vi "Target Logging.vi"(6 "rt fifo":refnum<k33>) -> (0 "Stop Loop":bool)   [LabVIEW 2018]
uses:
  Target Logging Cluster.ctl
  Target Sensors.ctl
  COBRA-Libraries/Data Logging/COBRA Logging and Loop Timing Library.lvlib
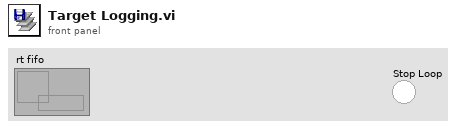
[diagram p1: front panel]
types:
  T1 = typedef "Target Logging Cluster.ctl" = cluster{"Valid for Logging?":bool, "Target Sensors":T2}
  T2 = typedef "Target Sensors.ctl" = cluster{"Raw Cable Force (N)":dbl, "Prosthesis Angle (deg)":dbl, "Main Clock Line (s)":dbl}
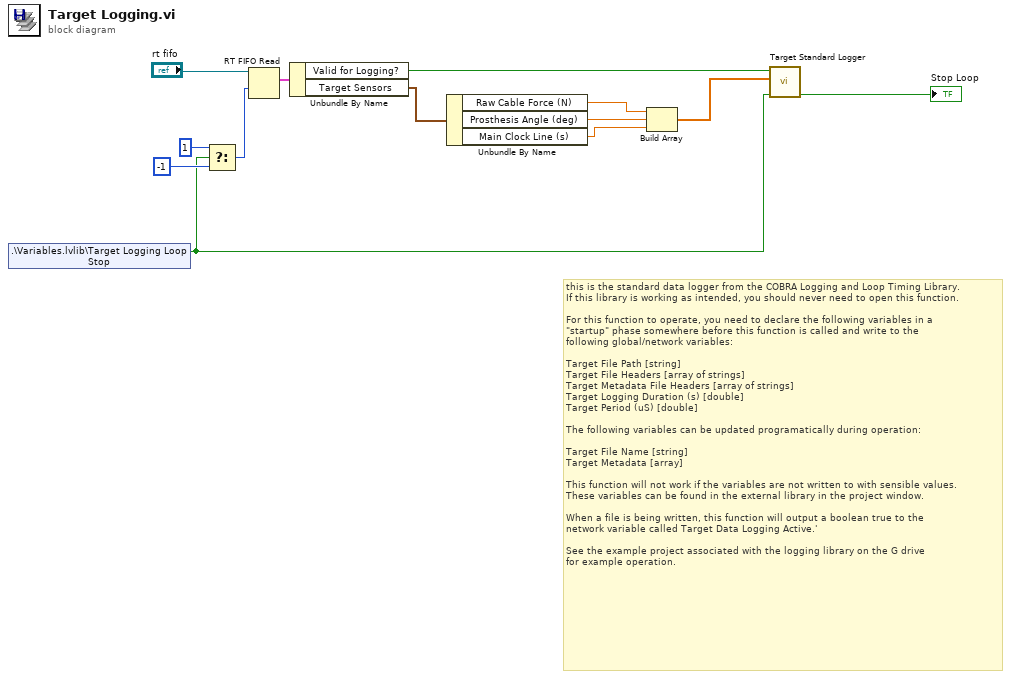
[diagram p0: block diagram]
diagram:
  # "this is the standard data logger from the COBRA Logging and Loop Timing Library.\nIf this library is working as intended, you should never need to open this function.\n\nFor this function to operate, you need to declare the following variables in a\n\"startup\" phase somewhere before this function is called and write to the\nfollowing global/network variables:\n\nTarget File Path [string]\nTarget File Headers [array of strings]\nTarget Metadata File Headers [array of strings]\nTarget Logging Duration (s) [double]\nTarget Period (uS) [double]\n\nThe following variables can be updated programatically during operation:\n\nTarget File Name [string]\nTarget Metadata [array]\n\nThis function will not work if the variables are not written to with sensible values.\nThese variables can be found in the external library in the project window.\n\nWhen a file is being written, this function will output a boolean true to the\nnetwork variable called Target Data Logging Active.'\n\nSee the example project associated with the logging library on the G drive\nfor example operation."
  n1 = shared-variable ".\\Variables.lvlib\\Target Logging Loop Stop"() -> (w1:bool)  [unwired: 1 in, 1 out]
  n2 = Select(t=1, s=w1, f=-1) -> (s? t:f=w11:i32)
  n3 = RT FIFO Read(0:"rt fifo", 2:w11) -> (9:w9:T1)  [unwired: 2 in, 4 out]
  n4 = Unbundle By Name(w9) -> ("Valid for Logging?"=w3:bool, "Target Sensors"=w8:T2)
  n5 = Unbundle By Name(w8) -> ("Raw Cable Force (N)"=w7:dbl, "Prosthesis Angle (deg)"=w6:dbl, "Main Clock Line (s)"=w5:dbl)
  n6 = Build Array(w7, w6, w5) -> (w2:dbl[])
  n7 = call "Target Standard Logger.vi"("Stop Command"=w1, "Incoming Data Array"=w2, "Valid for Logging?"=w3) -> ("Ok to Stop Logging Loop"=→"Stop Loop":bool)  [unwired: 8 in]
